vi "connect.vi"(8 "error in (no error)":errorcluster, 9 "TCP_IP.lvclass (in)":refnum<class "TCP_IP.lvclass">, 10 "IP address to listen on\n(blank to allow all networks)":string, 11 "port":u16=9000) -> (0 "error out":errorcluster, 1 "TCP_IP.lvclass":refnum<class "TCP_IP.lvclass">)   [LabVIEW 2014, in "TCP_IP.lvclass"]
uses:
  TCP_IP.lvclass
  Experiment/states.ctl
  TCP_IP.lvclass/TCP_IP.ctl
  Globals.vi
  Experiment/Experiment.lvclass
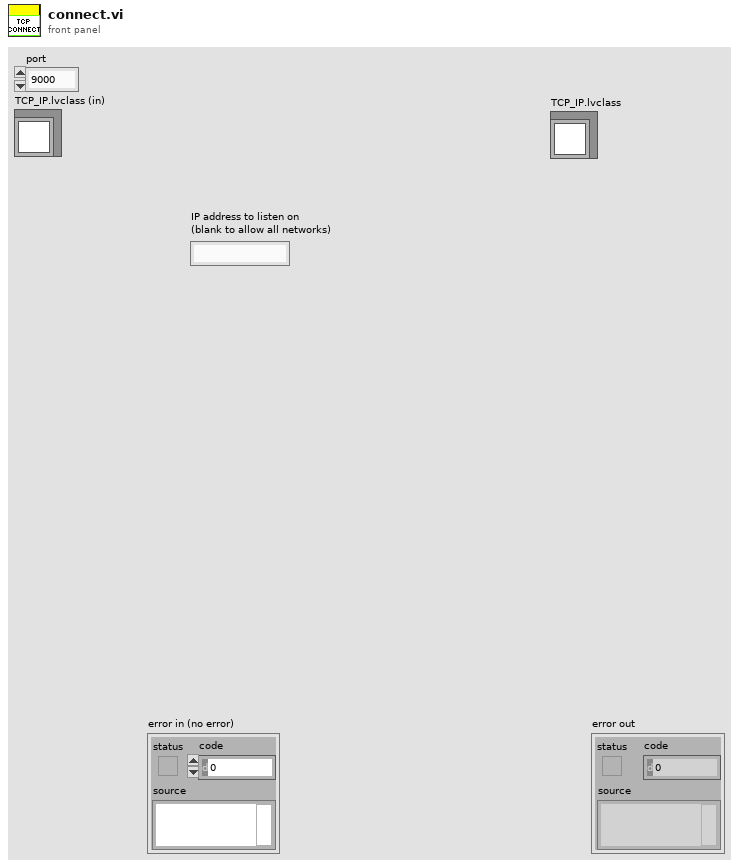
[diagram p1: front panel]
types:
  T1 = typedef "Experiment.lvclass/states.ctl" = enum16{"run", "pause", "shutdown gracefully", "halt immediately", "waiting for connection", "waiting for command"}
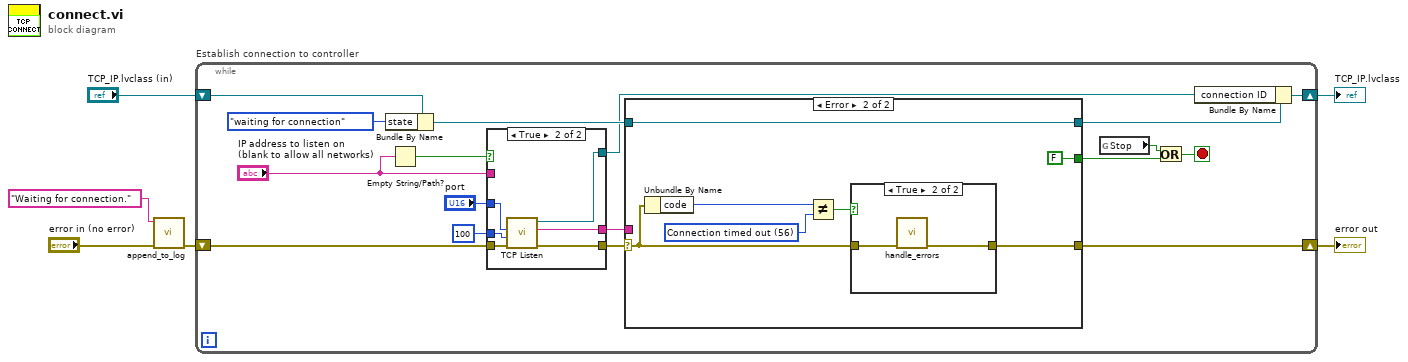
[diagram p0: block diagram]
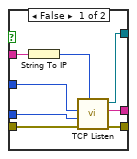
[diagram p2: hidden frame]
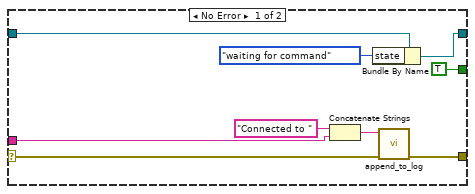
[diagram p3: hidden frame]
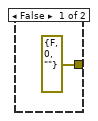
[diagram p4: hidden frame]
diagram:
  n1 = call "append_to_log.vi"("error in"="error in (no error)", "string"="Waiting for connection." ("Status")) -> ("error out"=w1:errorcluster)  [unwired: 9 in]
  n2 = while "Establish connection to controller" {
    shift-right: [w12] -> w5
    shift-left: "TCP_IP.lvclass (in)" -> [w16]
    shift-right: [w11] -> w4
    shift-left: w1 -> [w10]
    stop <- w18 stop-if-true
    n3 = Bundle By Name(cluster=w16, "state"=states."waiting for connection") -> (w15:refnum<class "TCP_IP.lvclass">)
    n4 = Empty String/Path?(string/path="IP address to listen on\n(blank to allow all networks)") -> (empty?=w8:bool)
    n5 = case shown="True" w8 {
      tunnel: 100 -> [w31 w35]
      tunnel: [w30 w33] -> w22
      tunnel: [w29 w36] -> w21
      tunnel: "port" -> [w28 w32]
      tunnel: [w27 w34] -> w14
      tunnel: w10 -> [w26 w37]
      tunnel: "IP address to listen on\n(blank to allow all networks)" -> [w24 _]
      frame False {
        n6 = String To IP(1:w24) -> (0:w25:u32)
        n7 = call <vilib>:"TCP Listen.vi"("net address"=w25, "error in (no error)"=w26, "timeout ms (wait forever: -1)"=w31, "port"=w28) -> ("error out"=w29:errorcluster, "remote address"=w30:string, "connection ID"=w27:refnum<k5>)  [unwired: 3 in, 2 out]
      }
      frame True {
        n8 = call <vilib>:"TCP Listen.vi"("error in (no error)"=w37, "timeout ms (wait forever: -1)"=w35, "port"=w32) -> ("error out"=w36:errorcluster, "remote address"=w33:string, "connection ID"=w34:refnum<k5>)  [unwired: 4 in, 2 out]
      }
    }
    n9 = case shown="Error" w21 {
      selector: w21 -> [w42 w50]
      tunnel: w22 -> [w45 _]
      tunnel: [TRUE FALSE] -> w19
      tunnel: w15 -> [w40 w48]
      tunnel: [w39 w48] -> w13
      tunnel: [w38 w47] -> w11
      frame No Error {
        n10 = Concatenate Strings("Connected to " ("string"), w45) -> (w44:string)
        n11 = Bundle By Name(cluster=w40, "state"=states."waiting for command") -> (w39:refnum<class "TCP_IP.lvclass">)
        n12 = call "append_to_log.vi"("error in"=w42, "string"=w44) -> ("error out"=w38:errorcluster)  [unwired: 9 in]
      }
      frame Error {
        w53 = 56 items=["No Error", "Argument Error", "Memory Full", "Out of Zone", "End of File", "File Already Open", "Generic File IO Error", "File Not Found", "File Permission Error", "Disk Full", "Duplicate Path", "Too Many Files Open", "Not Enabled", "Resource File Not Found", "Cannot Add Resource", "Resource Not Found", "Image Not Found", "Image Memory Error", "Pen Does Not Exist", "Config Bad Type", "Config Token Not Found", "Config Parse Error", "Config Memory Error", "Bad External Code Format", "Bad External Code Offset", "External Code Not Present", "Null Window", "Destroy Window Mixup", "Null Menu", "Print Aborted", "Bad Print Record", "Print Driver Error", "Windows Error During Print", "Memory Error During Print", "Print Dialog Error", "Generic Print Error", "Invalid Device Refnum", "Device Not Found", "Device Parameter Error", "Device Unit Error", "Can't Open Device", "Device Call Aborted", "Generic Error", "Cancelled By User", "Object ID Too Low", "Object ID Too High", "Object Not In Heap", "Unknown Heap", "Bad DefProc ID", "DefProc Not In Table", "Message Out Of Range", "Null Method", "Unknown Message", "Manager Call Not Supported", "Bad address", "Connection In progress", "Connection timed out", "Connection is already in progress", "Network attribute not supported", "Network error", "Address in use", "System out of memory", "Connection aborted", "Connection refused", "Connection is not connected", "Connection is already connected", "Connection closed", "Initialize error (interapplication manager)", "Bad occurrence", "Wait on unbound occurrence handler", "Occurrence queue overflow", "Bad path", "Semaphore not signaled", "Unrecognized type (interapplication manager)"] ("1st Error to Convert")
        n13 = Unbundle By Name(w50) -> ("code"=w52:i32)
        n14 = Not Equal?(x=w52, y=w53) -> (x != y?=w51:bool)
        n15 = case shown="True" w51 {
          tunnel: w50 -> [_ w56]
          tunnel: [errorcluster {"status"=FALSE, "code"=0, "source"=""} ("error out") w55] -> w47
          frame False {
          }
          frame True {
            n16 = call "handle_errors.vi"("error in (no error)"=w56) -> ("error out"=w55:errorcluster)  [unwired: 14 in]
          }
        }
      }
    }
    n17 = global read "Globals.vi" "Stop"() -> (w9:bool)
    n18 = Or(x=w9, y=w19) -> (x .or. y?=w18:bool)
    n19 = Bundle By Name(cluster=w13, "connection ID"=w14) -> (w12:refnum<class "TCP_IP.lvclass">)
  }
  "TCP_IP.lvclass" <- w5
  "error out" <- w4
